vi "Find Channel.vi"(8 "error in":errorcluster, 10 "channel name":string, 11 "channels":T1[](array[typedef]) {"core"."string offset" format="%d bytes"}) -> (0 "error out":errorcluster, 1 "found?":bool, 2 "channel index":i32, 3 "channels out":T1[](array[typedef]) {"core"."string offset" format="%d bytes"})   [LabVIEW 2020, in "DSF Configuration API.lvlib"]
uses:
  DSF Configuration API.lvlib
  Includes/DSF Core.lvlibp/Typedefs/DSF Settings Info.ctl
  Includes/DSF Core.lvlibp
  Includes/DSF Core.lvlibp/Typedefs/DSF Engine Channel Configuration.ctl
  Includes/DSF Core.lvlibp/Typedefs/Core Channel Configuration.ctl
  Includes/DSF Core.lvlibp/Classes/Configuration/Core/Channel/Channel Configuration.lvclass
  Includes/DSF Core.lvlibp/Typedefs/DSF Data Type.ctl
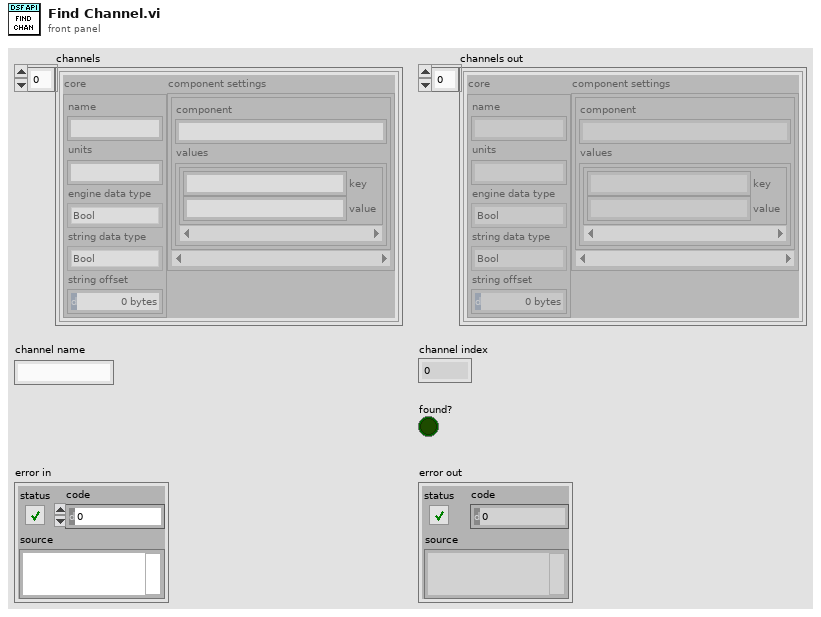
[diagram p1: front panel]
types:
  T1 = typedef "DSF Core.lvlibp/DSF Engine Channel Configuration.ctl" = cluster{"core":T2, "component settings":T4[]}
  T2 = typedef "DSF Core.lvlibp/Channel Configuration.lvclass/Core Channel Configuration.ctl" = cluster{"name":string, "units":string, "engine data type":T3, "string data type":T3, "string offset":u64}
  T3 = typedef "DSF Core.lvlibp/DSF Data Type.ctl" = enum8{"Bool", "SGL", "DBL", "I8", "I16", "I32", "I64", "U8", "U16", "U32", "U64"}
  T4 = typedef "DSF Core.lvlibp/DSF Settings Info.ctl" = cluster{"component":string, "values":cluster{"key":string, "value":string}[]}
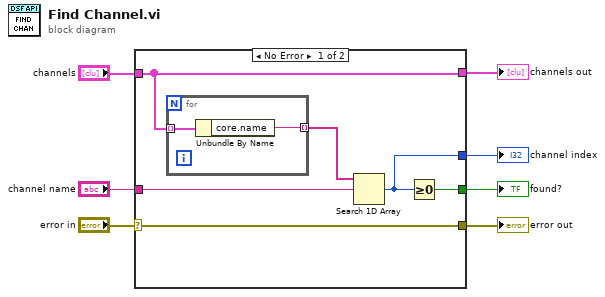
[diagram p0: block diagram]
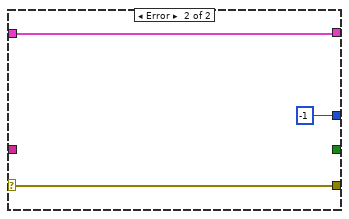
[diagram p2: hidden frame]
diagram:
  n1 = case shown="No Error" "error in" {
    selector: "error in" -> [w10 w18]
    tunnel: "channel name" -> [w13 _]
    tunnel: [w11 _] -> w6
    tunnel: [w10 w18] -> w4
    tunnel: [w9 -1 ("index of element")] -> w3
    tunnel: "channels" -> [w8 w16]
    tunnel: [w8 w16] -> w1
    frame No Error {
      n2 = for {
        tunnel: w8 -> [w15] mode=indexing
        tunnel: [w14] -> w12 mode=indexing
        n3 = Unbundle By Name(w15) -> ("core.name"=w14:string)
      }
      n4 = Search 1D Array(1D array=w12, element=w13) -> (index of element=w9:i32)  [unwired: 1 in]
      n5 = Greater Or Equal To 0?(x=w9) -> (x >= 0?=w11:bool)
    }
    frame Error {
    }
  }
  "found?" <- w6
  "error out" <- w4
  "channel index" <- w3
  "channels out" <- w1
